vi "AddTestMethod_Item_OnDblClick.vi"(11 "Object":T1) -> ()   [LabVIEW 2013]
uses:
  <resource>/Framework/Providers/API/ItemRef.ctl
panel:
  out "error out":errorcluster
  in  "error in":errorcluster
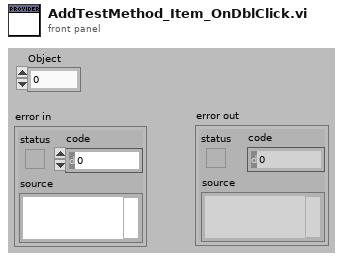
[diagram p1: front panel]
types:
  T1 = typedef "ItemRef.ctl" = u64
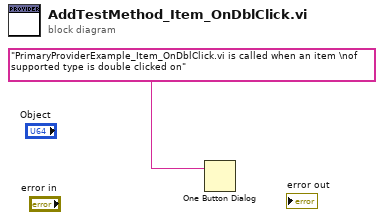
[diagram p0: block diagram]
diagram:
  n1 = One Button Dialog(message="PrimaryProviderExample_Item_OnDblClick.vi is called when an item \nof supported type is double clicked on") -> ()  [unwired: 1 in, 1 out]
